vi "IMU Stop.vi"() -> ()   [LabVIEW 2016]
panel:
  in  "IMU Stop":bool
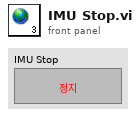
[diagram p1: front panel]
diagram:
